vi "Close.vi"(8 "error in (no error)":errorcluster, 11 "Network_Streams in":T1) -> (0 "error out":errorcluster)   [LabVIEW 2020, in "Communication VIs.lvlib" / "Network.lvlib"]
uses:
  Network.lvlib
  Network Streams.ctl
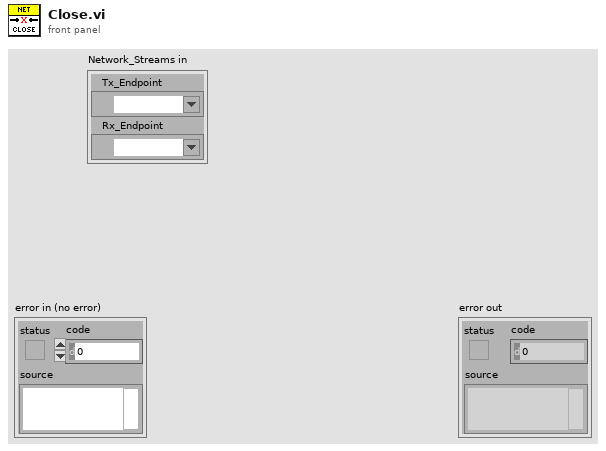
[diagram p1: front panel]
types:
  T1 = typedef "Communication VIs.lvlib/Network.lvlib/Network Streams.ctl" = cluster{"Tx_Endpoint":refnum<k21>, "Rx_Endpoint":refnum<k21>}
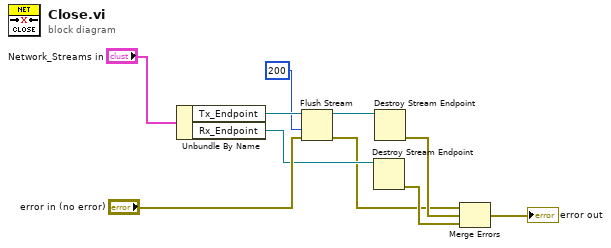
[diagram p0: block diagram]
diagram:
  n1 = Unbundle By Name("Network_Streams in") -> ("Tx_Endpoint"=w9:refnum<k21>, "Rx_Endpoint"=w5:refnum<k21>)
  n2 = Flush Stream(8:"error in (no error)", 9:200 ("timeout in ms (-1)"), 11:w9) -> (0:w3:errorcluster, 3:w8:refnum<k21>)  [unwired: 1 in, 1 out]
  n3 = Destroy Stream Endpoint(11:w5) -> (0:w4:errorcluster)  [unwired: 1 in]
  n4 = Destroy Stream Endpoint(11:w8) -> (0:w7:errorcluster)  [unwired: 1 in]
  n5 = Merge Errors(w3, w7, w4) -> (→"error out":errorcluster)
